vi "Config Spark Max Output HW Get Set.vi"(6 "Get(f) Set(t)":bool, 7 "SparkMax Output":T1, 8 "Error":errorcluster, 11 "Drive Refs":T3) -> (0 "Error Out":errorcluster, 3 "Drive Refs Out":T3, 5 "SparkMax Output Out":T1)   [LabVIEW 2023, in "Swerve-SteerSRX-DriveSpark-AbsAnalog_ACT.lvlib"]
uses:
  Swerve-SteerSRX-DriveSpark-AbsAnalog_ACT.lvlib
  <vilib>/Rock Robotics/WPI/MotorControl/WPI_MotorControlDeviceRef.ctl
  <vilib>/Rock Robotics/WPI/MotorControl/WPI_MotorControlType.ctl
  <vilib>/Rock Robotics/SystemInterfaces/DIO/FPGA_DIOPWMChannel.ctl
  <vilib>/Rock Robotics/WPI/PWM/WPI_PWMDeadband.ctl
  <vilib>/Rock Robotics/SystemInterfaces/DIO/FPGA_DIOChannel.ctl
  Shared Code/TypeDefs/Cluster_SparkMax Config_Motor Output.ctl
  <vilib>/Rock Robotics/WPI/ThirdParty/REV Robotics/REVLib/Typedef/Spark MAX Idle Mode.ctl
  <vilib>/Rock Robotics/WPI/ThirdParty/REV Robotics/REVLib/Typedef/Spark MAX Parameter ID.ctl
  <vilib>/Rock Robotics/WPI/ThirdParty/REV Robotics/REVLib/Typedef/Spark MAX Parameter Type.ctl
  <vilib>/Utility/error.llb/Trim Whitespace One-Sided.vi
  <vilib>/Rock Robotics/WPI/ThirdParty/REV Robotics/REVLib/SubVI/Private/Spark MAX Set Parameter dbl.vi
  <vilib>/Utility/Data Type/NI_Data Type.lvlib
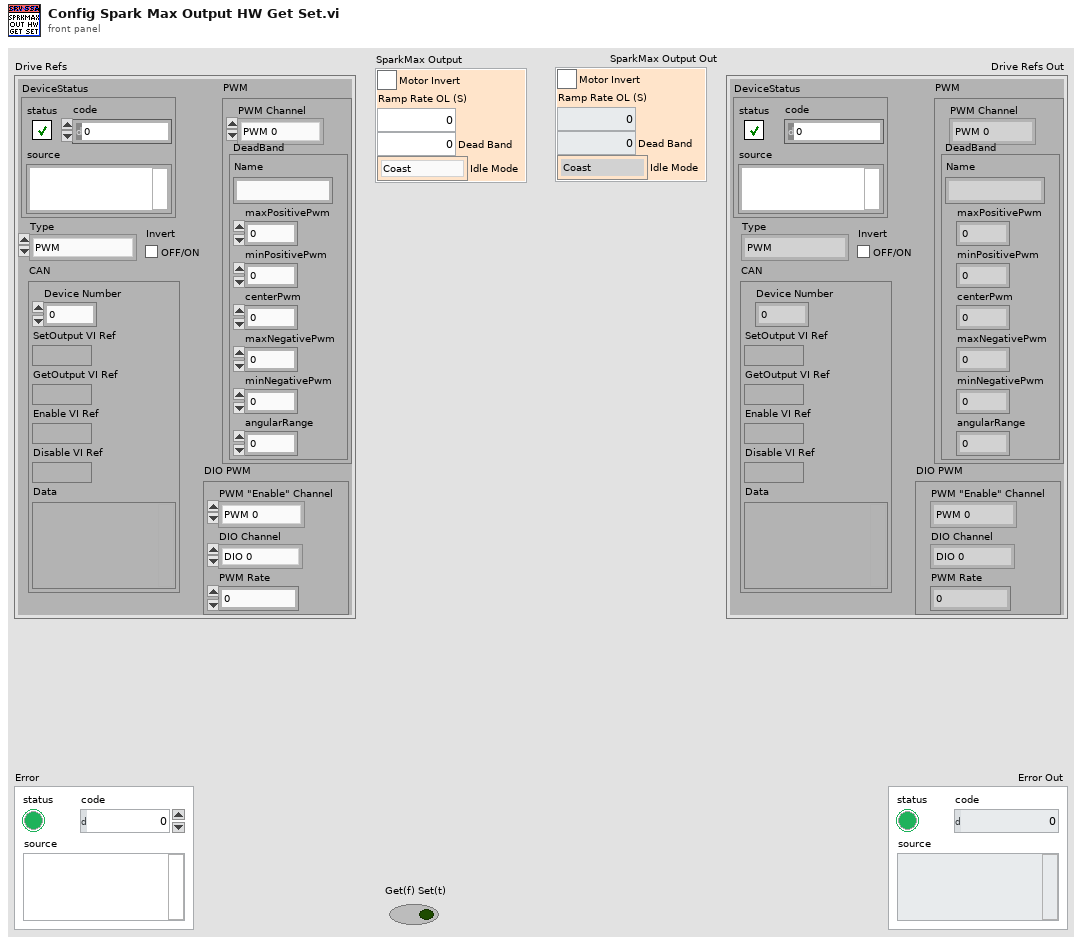
[diagram p1: front panel]
types:
  T1 = typedef "Cluster_SparkMax Config_Motor Output.ctl" = cluster{"Motor Invert":bool, "Ramp Rate OL (S)":dbl, "Dead Band":dbl, "Idle Mode":T2}
  T2 = typedef "Spark MAX Idle Mode.ctl" = enum16{"Coast", "Brake"}
  T3 = typedef "WPI_MotorControlDeviceRef.ctl" = cluster{"DeviceStatus":errorcluster, "Type":T4, "PWM":cluster{"PWM Channel":T5, "DeadBand":T6}, "CAN":cluster{"Device Number":u8, "SetOutput VI Ref":variant, "GetOutput VI Ref":variant, "Enable VI Ref":variant, "Disable VI Ref":variant, "Data":variant}, "Invert":bool, "DIO PWM":cluster{"PWM \"Enable\" Channel":T5, "DIOChannel":T7, "PWM Rate":dbl}}
  T4 = typedef "WPI_MotorControlType.ctl" = enum16{"PWM", "CAN", "DIO PWM"}
  T5 = typedef "FPGA_DIOPWMChannel.ctl" = enum8{"PWM 0", "PWM 1", "PWM 2", "PWM 3", "PWM 4", "PWM 5", "PWM 6", "PWM 7", "PWM 8", "PWM 9", "PWM MXP 0", "PWM MXP 1", "PWM MXP 2", "PWM MXP 3", "PWM MXP 4", "PWM MXP 5", "PWM MXP 6", "PWM MXP 7", "PWM MXP 8", "PWM MXP 9", "Invalid"}
  T6 = typedef "WPI_PWMDeadband.ctl" = cluster{"Name":string, "maxPositivePwm":i32, "minPositivePwm":i32, "centerPwm":i32, "maxNegativePwm":i32, "minNegativePwm":i32, "angularRange":u16}
  T7 = typedef "FPGA_DIOChannel.ctl" = enum8{"DIO 0", "DIO 1", "DIO 2", "DIO 3", "DIO 4", "DIO 5", "DIO 6", "DIO 7", "DIO 8", "DIO 9", "DIO MXP 0", "DIO MXP 1", "DIO MXP 2", "DIO MXP 3", "DIO MXP 4", "DIO MXP 5", "DIO MXP 6", "DIO MXP 7", "DIO MXP 8", "DIO MXP 9", "DIO MXP 10", "DIO MXP 11", "DIO MXP 12", "DIO MXP 13", "DIO MXP 14", "DIO MXP 15", "SPI Port CS1", "SPI Port CS2", "SPI Port CS3", "SPI Port MISO", "SPI Port MOSI", "Invalid"}
  T8 = typedef "Spark MAX Parameter ID.ctl" = enum16{"kCanID", "kInputMode", "kMotorType", "kCommAdvance", "kSensorType", "kCtrlType", "kIdleMode", "kInputDeadband", "kFeedbackSensorPID0", "kFeedbackSensorPID1", "kPolePairs", "kCurrentChop", "kCurrentChopCycles", "kP_0", "kI_0", "kD_0", "kF_0", "kIZone_0", "kDFilter_0", "kOutputMin_0", "kOutputMax_0", "kP_1", "kI_1", "kD_1", "kF_1", "kIZone_1", "kDFilter_1", "kOutputMin_1", "kOutputMax_1", "kP_2", "kI_2", "kD_2", "kF_2", "kIZone_2", "kDFilter_2", "kOutputMin_2", "kOutputMax_2", "kP_3", "kI_3", "kD_3", "kF_3", "kIZone_3", "kDFilter_3", "kOutputMin_3", "kOutputMax_3", "kInverted", "kOutputRatio", "kSerialNumberLow", "kSerialNumberMid", "kSerialNumberHigh", "kLimitSwitchFwdPolarity", "kLimitSwitchRevPolarity", "kHardLimitFwdEn", "kHardLimitRevEn", "kSoftLimitFwdEn", "kSoftLimitRevEn", "kRampRate", "kFollowerID", "kFollowerConfig", "kSmartCurrentStallLimit", "kSmartCurrentFreeLimit", "kSmartCurrentConfig", "kSmartCurrentReserved", "kMotorKv", "kMotorR", "kMotorL", "kMotorRsvd1", "kMotorRsvd2", "kMotorRsvd3", "kEncoderCountsPerRev", "kEncoderAverageDepth", "kEncoderSampleDelta", "kEncoderInverted", "kEncoderRsvd1", "kClosedLoopVoltageMode", "kCompensatedNominalVoltage", "kSmartMotionMaxVelocity_0", "kSmartMotionMaxAccel_0", "kSmartMotionMinVelOutput_0", "kSmartMotionAllowedClosedLoopError_0", "kSmartMotionAccelStrategy_0", "kSmartMotionMaxVelocity_1", "kSmartMotionMaxAccel_1", "kSmartMotionMinVelOutput_1", "kSmartMotionAllowedClosedLoopError_1", "kSmartMotionAccelStrategy_1", "kSmartMotionMaxVelocity_2", "kSmartMotionMaxAccel_2", "kSmartMotionMinVelOutput_2", "kSmartMotionAllowedClosedLoopError_2", "kSmartMotionAccelStrategy_2", "kSmartMotionMaxVelocity_3", "kSmartMotionMaxAccel_3", "kSmartMotionMinVelOutput_3", "kSmartMotionAllowedClosedLoopError_3", "kSmartMotionAccelStrategy_3", "kIMaxAccum_0", "kSlot3Placeholder1_0", "kSlot3Placeholder2_0", "kSlot3Placeholder3_0", "kIMaxAccum_1", "kSlot3Placeholder1_1", "kSlot3Placeholder2_1", "kSlot3Placeholder3_1", "kIMaxAccum_2", "kSlot3Placeholder1_2", "kSlot3Placeholder2_2", "kSlot3Placeholder3_2", "kIMaxAccum_3", "kSlot3Placeholder1_3", "kSlot3Placeholder2_3", "kSlot3Placeholder3_3", "kPositionConversionFactor", "kVelocityConversionFactor", "kClosedLoopRampRate", "kSoftLimitFwd", "kSoftLimitRev", "kSoftLimitRsvd0", "kSoftLimitRsvd1", "kAnalogPositionConversion", "kAnalogVelocityConversion", "kAnalogAverageDepth", "kAnalogSensorMode", "kAnalogInverted", "kAnalogSampleDelta", "kAnalogRsvd0", "kAnalogRsvd1", "kDataPortConfig", "kAltEncoderCountsPerRev", "kAltEncoderAverageDepth", "kAltEncoderSampleDelta", "kAltEncoderInverted", "kAltEncoderPositionConversion", "kAltEncoderVelocityConversion", "kAltEncoderRsvd0", "kAltEncoderRsvd1", "kHallSensorSampleRate", "kHallSensorAverageDepth", "kNumParameters", "kDutyCyclePositionFactor", "kDutyCycleVelocityFactor", "kDutyCycleInverted", "kDutyCycleSensorMode", "kDutyCycleAverageDepth", "kDutyCycleSampleDelta", "kDutyCycleOffsetv1p6p2", "kDutyCycleRsvd0", "kDutyCycleRsvd1", "kDutyCycleRsvd2", "kPositionPIDWrapEnable", "kPositionPIDMinInput", "kPositionPIDMaxInput", "kDutyCycleZeroCentered", "kDutyCyclePrescalar", "kDutyCycleOffset", "kProductId", "kDeviceMajorVersion", "kDeviceMinorVersion"}
  T9 = typedef "Spark MAX Parameter Type.ctl" = enum16{"Signed Int", "Unsigned Int", "Float", "Bool"}
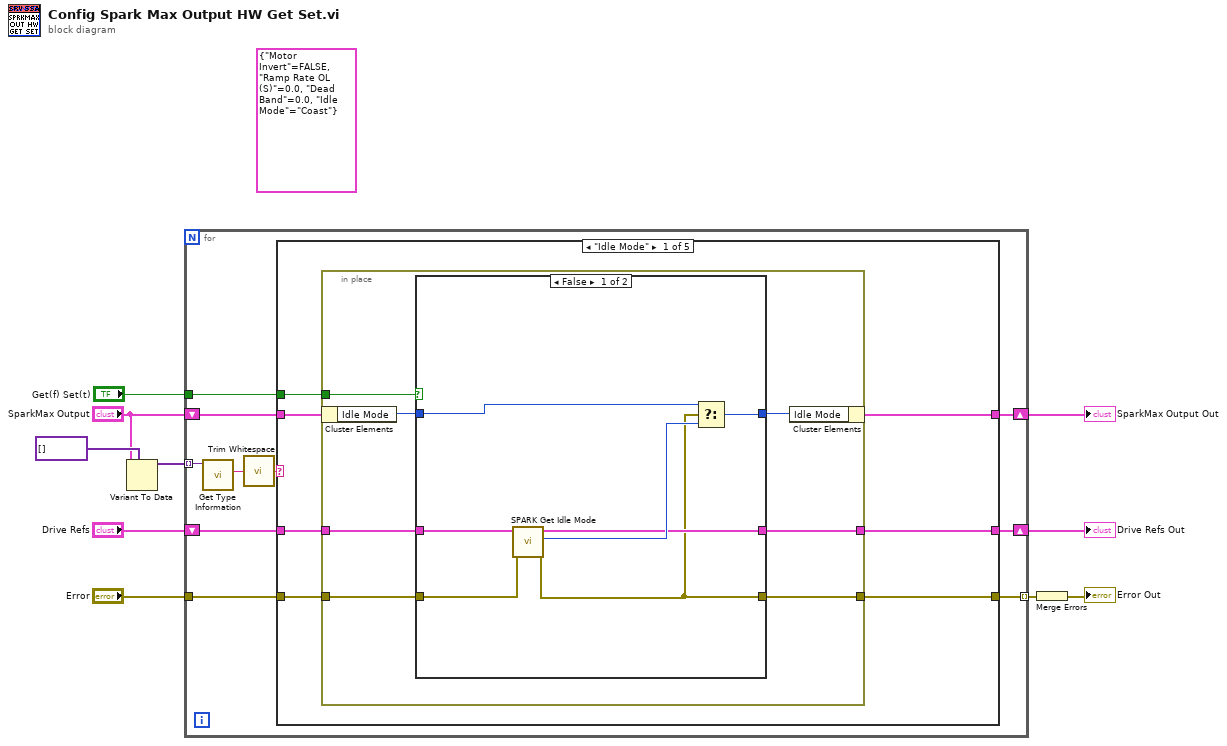
[diagram p0: block diagram]
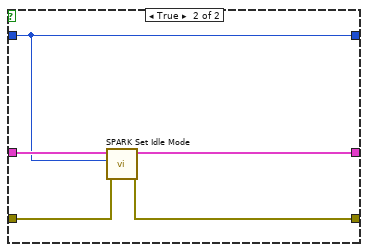
[diagram p2: hidden frame]
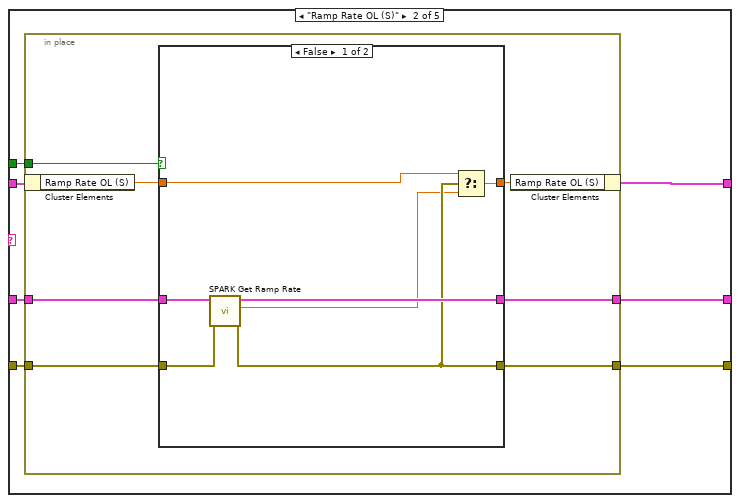
[diagram p3: hidden frame]
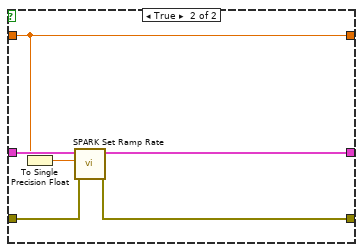
[diagram p4: hidden frame]
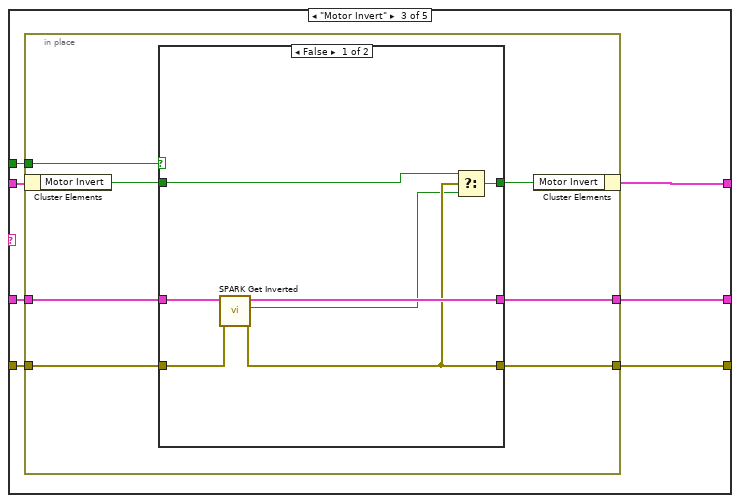
[diagram p5: hidden frame]
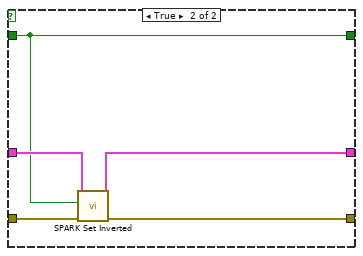
[diagram p6: hidden frame]
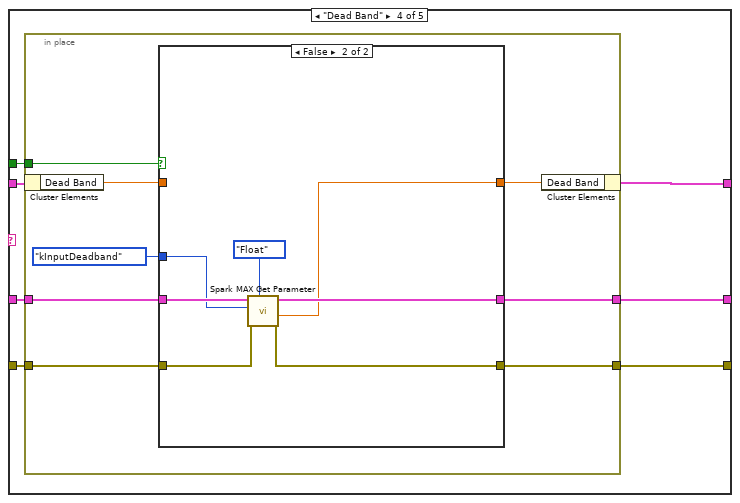
[diagram p7: hidden frame]
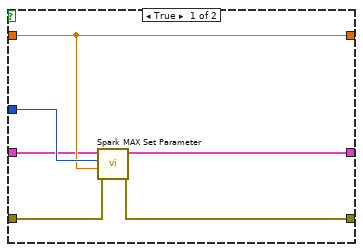
[diagram p8: hidden frame]
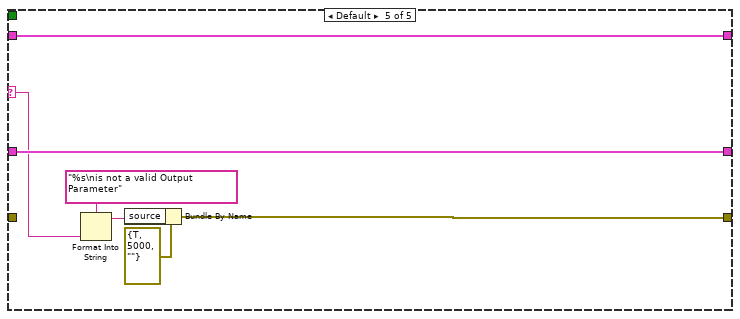
[diagram p9: hidden frame]
diagram:
  (unwired) T1 {"Motor Invert"=FALSE, "Ramp Rate OL (S)"=0.0, "Dead Band"=0.0, "Idle Mode"=enum."Coast"} ("SparkMax Output")
  n1 = Variant To Data(type=variant[] [], Variant="SparkMax Output") -> (data=w5:variant[])  [unwired: 1 in, 1 out]
  n2 = for {
    shift-right: [w11] -> w10
    shift-left: "SparkMax Output" -> [w17]
    shift-right: [w12] -> w8
    shift-left: "Drive Refs" -> [w16]
    tunnel: "Get(f) Set(t)" -> [w15]
    tunnel: w5 -> [w19] mode=indexing
    tunnel: "Error" -> [w14]
    tunnel: [w13] -> w2 mode=indexing
    n3 = call <vilib>:"Get Type Information.vi"("variant"=w19) -> ("name"=w20:string)  [unwired: 6 in, 4 out]
    n4 = call <vilib>:"Trim Whitespace.vi"("string"=w20) -> ("trimmed string"=w18:string)  [unwired: 1 in]
    n5 = case shown="\"Idle Mode\"" w18 {
      selector: w18 -> [_ _ _ _ w132]
      tunnel: w17 -> [w27 w53 w80 w106 w134]
      tunnel: w16 -> [w23 w49 w76 w102 w133]
      tunnel: w15 -> [w26 w52 w79 w105 _]
      tunnel: w14 -> [w25 w51 w78 w104 _]
      tunnel: [w24 w50 w77 w103 w130] -> w13
      tunnel: [w22 w48 w75 w101 w133] -> w12
      tunnel: [w21 w47 w74 w100 w134] -> w11
      frame "Idle Mode" {
        n6 = in-place {
          in-place-border: w26 -> [w34]
          in-place-border: w25 -> [w32]
          in-place-border: [w31] -> w24
          in-place-border: w23 -> [w30]
          in-place-border: [w29] -> w22
          n7 = in-place-cluster #1(w27) -> ("Idle Mode"=w33:T2)
          n8 = case shown="False" w34 {
            tunnel: w33 -> [w41 w44]
            tunnel: w32 -> [w36 w43]
            tunnel: [w35 w42] -> w31
            tunnel: w30 -> [w37 w46]
            tunnel: [w38 w45] -> w29
            tunnel: [w40 w44] -> w28
            frame False {
              n9 = call <vilib>:"SPARK Get Idle Mode.vi"("error in (no error)"=w36, "MotorControlDeviceRef in"=w37) -> ("error out"=w35:errorcluster, "Idle Mode"=w39:T2, "MotorControlDeviceRef out"=w38:T3)  [unwired: 7 in]
              n10 = Select(t=w41, s=w35, f=w39) -> (s? t:f=w40:T2)
            }
            frame True {
              n11 = call <vilib>:"SPARK Set Idle Mode.vi"("error in (no error)"=w43, "Idle Mode"=w44, "MotorControlDeviceRef in"=w46) -> ("error out"=w42:errorcluster, "MotorControlDeviceRef out"=w45:T3)  [unwired: 7 in]
            }
          }
          n12 = in-place-cluster #1("Idle Mode"=w28) -> (w21:T1)
        }
      }
      frame "Ramp Rate OL (S)" {
        n13 = in-place {
          in-place-border: w52 -> [w60]
          in-place-border: w51 -> [w58]
          in-place-border: [w57] -> w50
          in-place-border: w49 -> [w56]
          in-place-border: [w55] -> w48
          n14 = in-place-cluster #2(w53) -> ("Ramp Rate OL (S)"=w59:dbl)
          n15 = case shown="False" w60 {
            tunnel: w59 -> [w67 w69]
            tunnel: w58 -> [w63 w70]
            tunnel: [w62 w71] -> w57
            tunnel: w56 -> [w65 w73]
            tunnel: [w64 w72] -> w55
            tunnel: [w66 w69] -> w54
            frame False {
              n16 = call <vilib>:"SPARK Get Ramp Rate.vi"("error in (no error)"=w63, "MotorControlDeviceRef in"=w65) -> ("error out"=w62:errorcluster, "Ramp Rate"=w61:dbl, "MotorControlDeviceRef out"=w64:T3)  [unwired: 7 in]
              n17 = Select(t=w67, s=w62, f=w61) -> (s? t:f=w66:dbl)
            }
            frame True {
              n18 = To Single Precision Float(number=w69) -> (single precision float=w68:sgl)
              n19 = call <vilib>:"SPARK Set Ramp Rate.vi"("error in (no error)"=w70, "Seconds from neutral to full (0)"=w68, "MotorControlDeviceRef in"=w73) -> ("error out"=w71:errorcluster, "MotorControlDeviceRef"=w72:T3)  [unwired: 7 in]
            }
          }
          n20 = in-place-cluster #2("Ramp Rate OL (S)"=w54) -> (w47:T1)
        }
      }
      frame "Motor Invert" {
        n21 = in-place {
          in-place-border: w79 -> [w87]
          in-place-border: w78 -> [w85]
          in-place-border: [w84] -> w77
          in-place-border: w76 -> [w83]
          in-place-border: [w82] -> w75
          n22 = in-place-cluster #3(w80) -> ("Motor Invert"=w86:bool)
          n23 = case shown="False" w87 {
            tunnel: w86 -> [w94 w95]
            tunnel: w85 -> [w90 w96]
            tunnel: [w89 w97] -> w84
            tunnel: w83 -> [w91 w99]
            tunnel: [w92 w98] -> w82
            tunnel: [w93 w95] -> w81
            frame False {
              n24 = call <vilib>:"SPARK Get Inverted.vi"("error in (no error)"=w90, "MotorControlDeviceRef in"=w91) -> ("error out"=w89:errorcluster, "Inverted"=w88:bool, "MotorControlDeviceRef out"=w92:T3)  [unwired: 7 in]
              n25 = Select(t=w94, s=w89, f=w88) -> (s? t:f=w93:bool)
            }
            frame True {
              n26 = call <vilib>:"SPARK Set Inverted.vi"("error in (no error)"=w96, "Inverted (F)"=w95, "MotorControlDeviceRef in"=w99) -> ("error out"=w97:errorcluster, "MotorControlDeviceRef out"=w98:T3)  [unwired: 7 in]
            }
          }
          n27 = in-place-cluster #3("Motor Invert"=w81) -> (w74:T1)
        }
      }
      frame "Dead Band" {
        n28 = in-place {
          in-place-border: w105 -> [w114]
          in-place-border: w104 -> [w112]
          in-place-border: [w111] -> w103
          in-place-border: w102 -> [w110]
          in-place-border: [w109] -> w101
          n29 = in-place-cluster #4(w106) -> ("Dead Band"=w113:dbl)
          n30 = case shown="False" w114 {
            tunnel: w113 -> [w119 _]
            tunnel: w112 -> [w116 w124]
            tunnel: [w115 w123] -> w111
            tunnel: w110 -> [w118 w126]
            tunnel: [w117 w125] -> w109
            tunnel: [w119 w121] -> w108
            tunnel: Spark_MAX_Parameter_ID."kInputDeadband" ("Parameter ID") -> [w120 w122]
            frame True {
              n31 = call-poly <vilib>:"Spark MAX Set Parameter.vi"("error in (no error)"=w116, "double precision float"=w119, "Parameter ID"=w120, "MotorControlDeviceRef"=w118) -> ("error out"=w115:errorcluster, "MotorControlDeviceRef"=w117:T3)  [unwired: 6 in]
            }
            frame False {
              n32 = call <vilib>:"Spark MAX Get Parameter.vi"("Expected Type"=Spark_MAX_Parameter_Type."Float", "error in (no error)"=w124, "Parameter ID in"=w122, "MotorControlDeviceRef in"=w126) -> ("error out"=w123:errorcluster, "float"=w121:dbl, "MotorControlDeviceRef"=w125:T3)  [unwired: 2 in, 3 out]
            }
          }
          n33 = in-place-cluster #4("Dead Band"=w108) -> (w100:T1)
        }
      }
      frame Default {
        n34 = Format Into String(format string="%s\nis not a valid Output Parameter", w132) -> (resulting string=w128:string)  [unwired: 2 in, 1 out]
        n35 = Bundle By Name(cluster=errorcluster {"status"=TRUE, "code"=5000, "source"=""} ("error out"), "source"=w128) -> (w130:errorcluster)
      }
    }
  }
  "Drive Refs Out" <- w8
  "SparkMax Output Out" <- w10
  n36 = Merge Errors(w2) -> (→"Error Out":errorcluster)
